vi "Read One Config Key.vi"(8 "error in (no error)":cluster{"状态":bool, "代码":i32, "源":string} caption="错误输入（无错误）", 9 "键":string, 10 "默认值":string, 11 "引用句柄输入":T1) -> (0 "error out":cluster{"状态":bool, "代码":i32, "源":string} caption="错误输出", 2 "值":string, 3 "引用句柄输出":T1)   [LabVIEW 2015, in "Air Cooler Application.lvlib" / "Air Cooler Application.lvclass"]
doc: "从配置文件中读取一个键。"
uses:
  Air Cooler Application.lvclass
  <vilib>/Utility/config.llb/Config Data RefNum.ctl
  <vilib>/Utility/config.llb/Read Key (String).vi
  <vilib>/Utility/config.llb/NI_LVConfig.lvlib
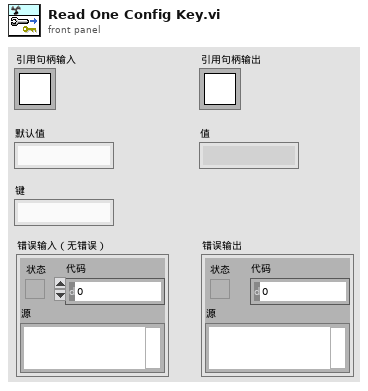
[diagram p1: front panel]
types:
  T1 = typedef "NI_LVConfig.lvlib/Config Data RefNum.ctl" = refnum<k1>
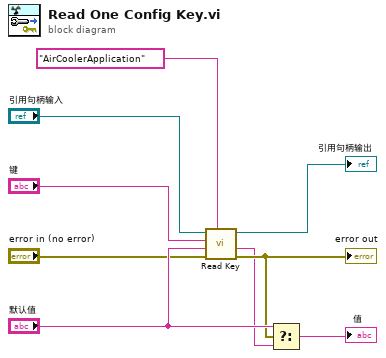
[diagram p0: block diagram]
diagram:
  n1 = call-poly <vilib>:"Read Key.vi"("section"="AirCoolerApplication", "error in (no error)"="error in (no error)", "default value"="默认值", "key"="键", "refnum"="引用句柄输入") -> ("error out"=w6:errorcluster, "value"=w4:string, "refnum out"=→"引用句柄输出":T1)  [unwired: 3 in, 1 out]
  "error out" <- w6
  n2 = Select(t="默认值", s=w6, f=w4) -> (s? t:f=→"值":string)
